vi "Add To Slack Demo (.NET).vi"() -> ()   [LabVIEW 2020]
uses:
  D:/Development/Standalone Diagnostics/Backend/SlackAPI/bin/Release/SlackAPI.dll
  Standalone Diagnostics/Backend/SlackAPI/bin/Release/SlackAPI.dll
panel:
  out "ToString":string
  in  "client_secret":string="f1e341df902b360dfbc2bfcae092b542"
  in  "client_id":string="1023330033985.1045128173975"
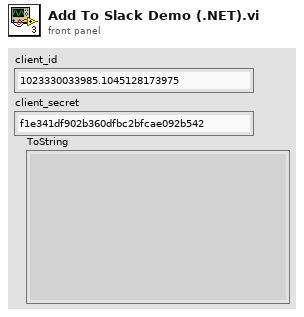
[diagram p1: front panel]
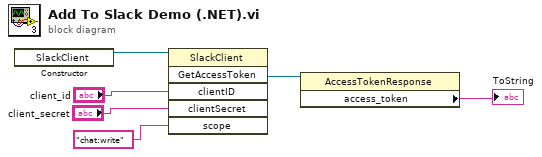
[diagram p0: block diagram]
diagram:
  n1 = constructor class="SlackClient"() -> (reference out=w6:refnum<k24>)  [unwired: 3 in, 2 out]
  n2 = invoke class="SlackClient" method="GetAccessToken"(reference=w6, "clientID"="client_id", "clientSecret"="client_secret", "scope"="chat:write") -> ("GetAccessToken"=w2:refnum<k24>)  [unwired: 2 in, 5 out]
  n3 = property class="AccessTokenResponse"(reference=w2) -> ("access_token"=→"ToString":string)  [unwired: 1 in, 2 out]
